vi "MSEncoder SubVI WfmCodeGen_AmpScan_Timestamp2WfmCode.vi"(7 "Parameters":T1, 8 "error in":errorcluster, 9 "Timeindex queue in":refnum<queue>, 10 "Display queue":refnum<queue>, 11 "WfmCode queue in":refnum<queue>) -> (0 "error out":errorcluster)   [LabVIEW 2018, in "MSEncoder.lvclass"]
uses:
  MSEncoder.lvclass
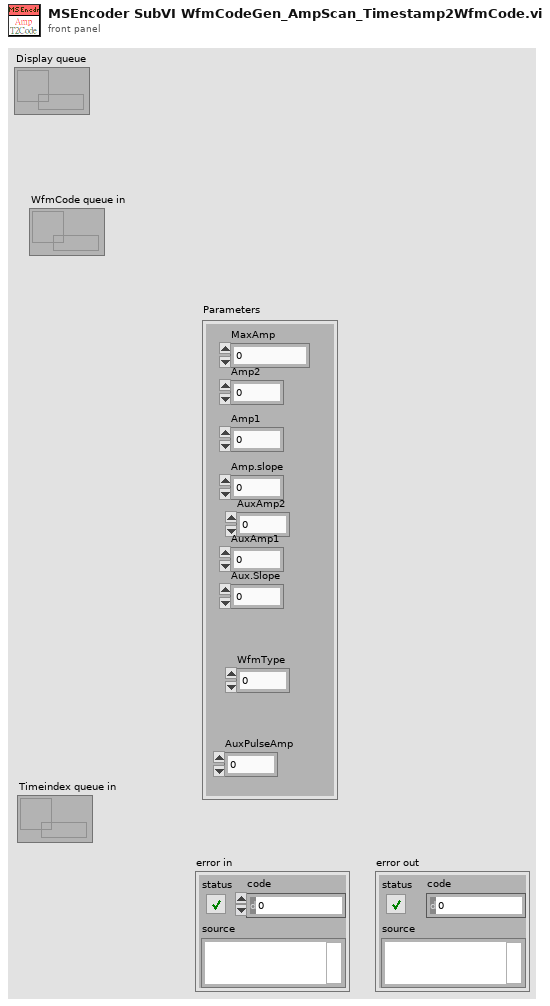
[diagram p1: front panel]
types:
  T1 = cluster{"MaxAmp":dbl, "Amp2":ext, "Amp1":ext, "Amp.slope":ext, "AuxAmp2":ext, "AuxAmp1":ext, "Aux.Slope":ext, "WfmType":u8, "AuxPulseAmp":u32}
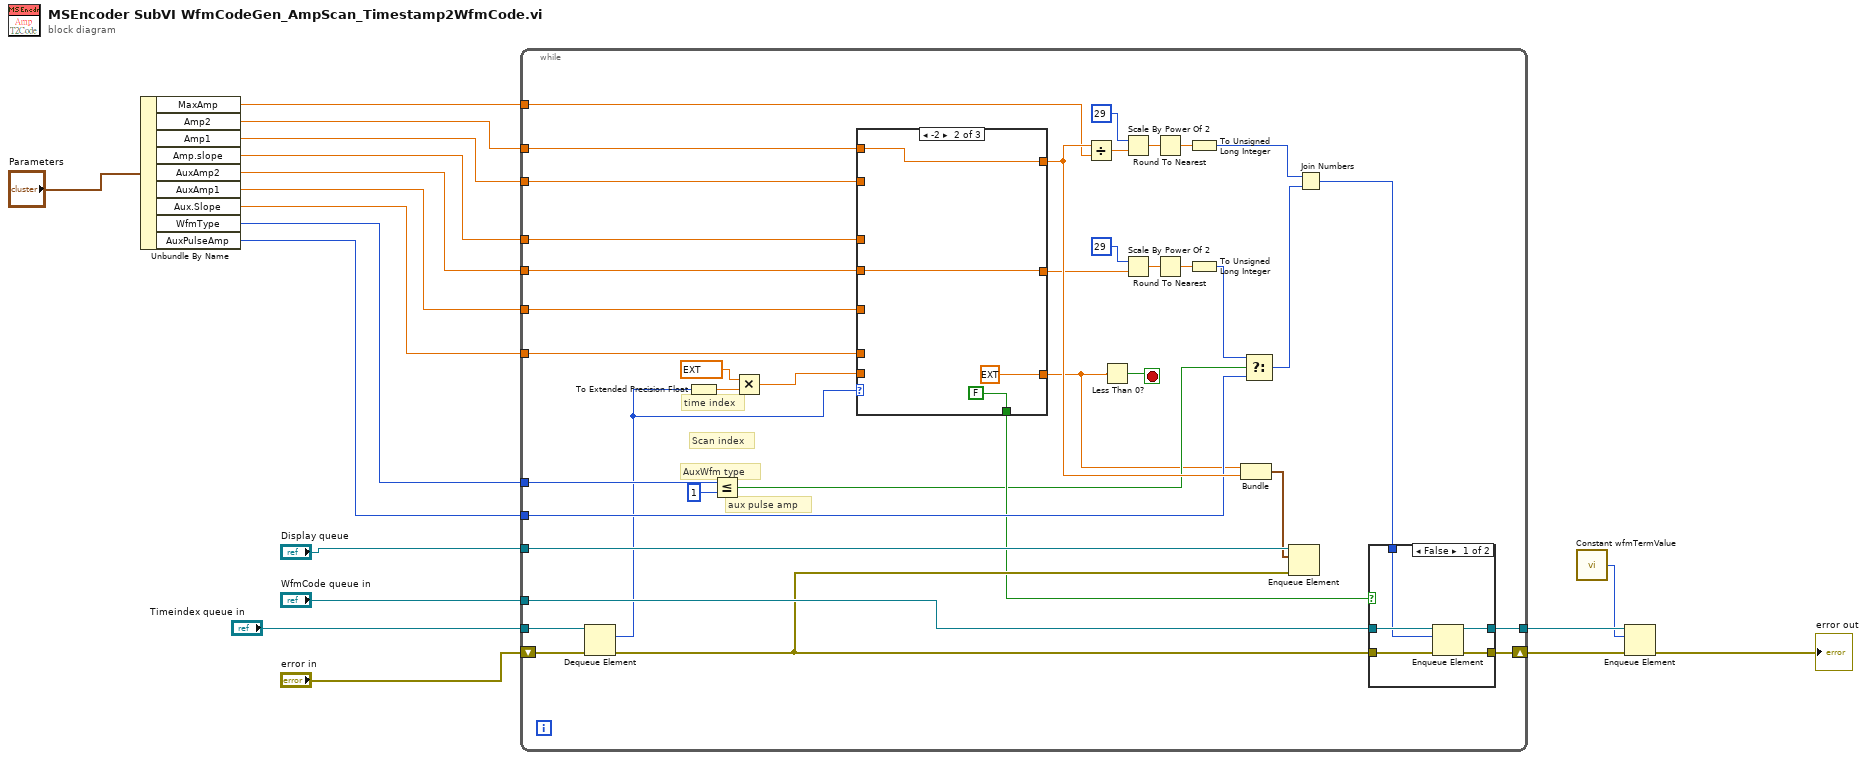
[diagram p0: block diagram]
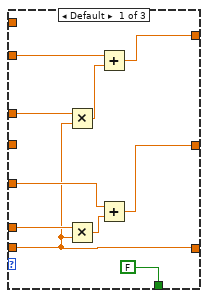
[diagram p3: hidden frame]
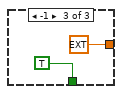
[diagram p4: hidden frame]
diagram:
  n1 = Unbundle By Name("Parameters") -> ("MaxAmp"=w16:dbl, "Amp2"=w15:ext, "Amp1"=w14:ext, "Amp.slope"=w13:ext, "AuxAmp2"=w12:ext, "AuxAmp1"=w11:ext, "Aux.Slope"=w10:ext, "WfmType"=w9:u8, "AuxPulseAmp"=w8:u32)
  n2 = while {
    tunnel: "WfmCode queue in" -> [w55]
    tunnel: "Display queue" -> [w54]
    tunnel: w16 -> [w37]
    tunnel: w15 -> [w36]
    tunnel: w14 -> [w35]
    tunnel: w13 -> [w34]
    tunnel: w12 -> [w33]
    tunnel: w11 -> [w32]
    tunnel: w10 -> [w31]
    tunnel: w9 -> [w30]
    tunnel: w8 -> [w29]
    tunnel: "Timeindex queue in" -> [w25]
    shift-right: [w57] -> w4
    shift-left: "error in" -> [w27]
    tunnel: [w22] -> w5
    stop <- w20 stop-if-true
    # "aux pulse amp"
    # "AuxWfm type"
    # "Scan index"
    # "time index"
    n3 = Dequeue Element(queue=w25, error in (no error)=w27) -> (element=w28:i64, error out=w26:errorcluster)  [unwired: 1 in, 2 out]
    n4 = To Extended Precision Float(1:w28) -> (0:w52:ext)
    n5 = Less Or Equal?(x=w30, y=u8 1) -> (x <= y?=w21:bool)
    n6 = Multiply(x=ext 2.5e-08, y=w52) -> (x*y=w39:ext)
    n7 = case shown="-2" w28 {
      tunnel: [w71 w78 _] -> w56
      tunnel: w36 -> [_ w78 _]
      tunnel: w35 -> [w73 _ _]
      tunnel: w34 -> [w72 _ _]
      tunnel: w39 -> [w65 _ _]
      tunnel: w31 -> [w70 _ _]
      tunnel: w32 -> [w68 _ _]
      tunnel: w33 -> [_ w77 _]
      tunnel: [w67 w77 _] -> w44
      tunnel: [FALSE FALSE TRUE] -> w24
      tunnel: [w65 ext -2.0 ext -1.0] -> w19
      frame Default {
        n8 = Multiply(x=w72, y=w65) -> (x*y=w74:ext)
        n9 = Multiply(x=w70, y=w65) -> (x*y=w69:ext)
        n10 = Add(x=w73, y=w74) -> (x+y=w71:ext)
        n11 = Add(x=w68, y=w69) -> (x+y=w67:ext)
      }
      frame -2 {
      }
      frame -1 {
      }
    }
    n12 = Divide(x=w56, y=w37) -> (x/y=w51:ext)
    n13 = Less Than 0?(x=w19) -> (x < 0?=w20:bool)
    n14 = Scale By Power Of 2(n=i16 29, x=w51) -> (x*2^n=w49:ext)
    n15 = Scale By Power Of 2(n=i16 29, x=w44) -> (x*2^n=w46:ext)
    n16 = Round To Nearest(number=w49) -> (nearest integer value=w48:ext)
    n17 = Round To Nearest(number=w46) -> (nearest integer value=w47:ext)
    n18 = To Unsigned Long Integer(number=w48) -> (unsigned 32bit integer=w43:u32)
    n19 = To Unsigned Long Integer(number=w47) -> (unsigned 32bit integer=w41:u32)
    n20 = Bundle(w19, "Amp2"=w56) -> (w23:cluster{ext, "Amp2":ext})  [unwired: 1 in]
    n21 = Select(t=w41, s=w21, f=w29) -> (s? t:f=w40:u32)
    n22 = Enqueue Element(queue=w54, element=w23, error in (no error)=w26) -> ()  [unwired: 1 in, 3 out]
    n23 = Join Numbers(hi=w43, lo=w40) -> ((hi.lo)=w38:u64)
    n24 = case shown="False" w24 {
      tunnel: w55 -> [w62 w64]
      tunnel: w26 -> [w61 w63]
      tunnel: [w60 w64] -> w22
      tunnel: [w59 w63] -> w57
      tunnel: w38 -> [w58 _]
      frame False {
        n25 = Enqueue Element(queue=w62, element=w58, error in (no error)=w61) -> (queue out=w60:refnum<queue>, error out=w59:errorcluster)  [unwired: 1 in, 1 out]
      }
      frame True {
      }
    }
  }
  n26 = call "Constant wfmTermValue.vi"() -> ("wfm end value"=w3:u64)
  n27 = Enqueue Element(queue=w5, element=w3, error in (no error)=w4) -> (error out=→"error out":errorcluster)  [unwired: 1 in, 2 out]
